vi "Default Success Response.vi"(8 "error in (no error)":errorcluster, 9 "Session In":refnum<class "Session.lvclass">, 10 "User":refnum<class "User.lvclass">) -> (0 "error out":errorcluster, 1 "Session":refnum<class "Session.lvclass">, 2 "Response":refnum<class "Response.lvclass">)   [LabVIEW 2020, in "HTTP Server.lvlib" / "Authentication Provider.lvclass"]
uses:
  Authentication Provider.lvclass
  lv-http-util/HTTP Utils/Response/Response.lvclass
  Session/Session.lvclass
  User/User.lvclass
  lv-http-util/HTTP Utils/Redirect Response/Redirect Response.lvclass
  C:/dev/lv20CE/relink/lv-http-util/HTTP Utils/Response/Response.lvclass
  lv-uri/URI/URI/URI.lvclass
  C:/dev/lv20CE/relink/lv-http-util/HTTP Utils/Redirect Response/Redirect Response.lvclass
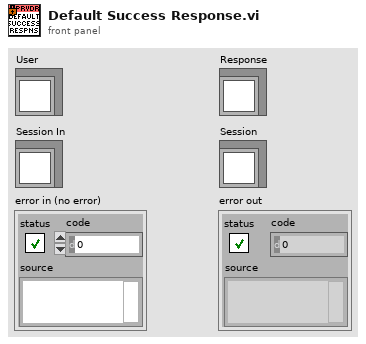
[diagram p1: front panel]
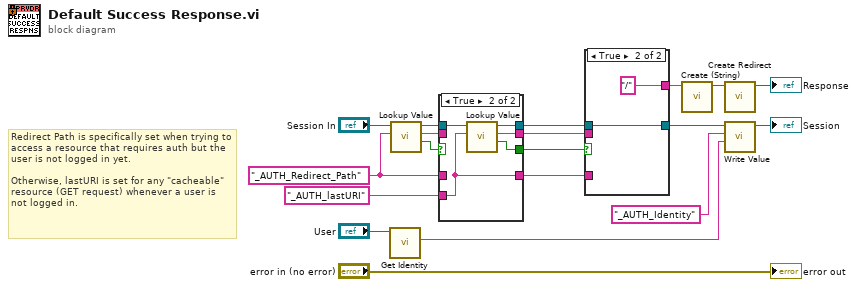
[diagram p0: block diagram]
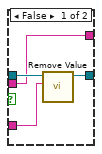
[diagram p2: hidden frame]
diagram:
  w7 = "_AUTH_Redirect_Path" ("Name")
  # "Redirect Path is specifically set when trying to access a resource that requires auth but the user is not logged in yet.\n\nOtherwise, lastURI is set for any \"cacheable\" resource (GET request) whenever a user is not logged in."
  n1 = call-dynamic "Get Identity.vi"("User in"="User") -> ("Identity"=w17:string)  [unwired: 8 in, 2 out]
  n2 = call "Lookup Value.vi"("Name"=w7, "Session in"="Session In") -> ("Not Found?"=w14:bool, "Value"=w12:string, "Session out"=w13:refnum<class "Session.lvclass">)  [unwired: 6 in, 1 out]
  n3 = case shown="True" w14 {
    tunnel: "_AUTH_lastURI" -> [_ w23]
    tunnel: w13 -> [w22 w27]
    tunnel: w12 -> [w21 _]
    tunnel: [_ w26] -> w9
    tunnel: [w21 w25] -> w10
    tunnel: [w22 w24] -> w11
    tunnel: [w20 w23] -> w8
    tunnel: w7 -> [w20 _]
    frame False {
    }
    frame True {
      n4 = call "Lookup Value.vi"("Name"=w23, "Session in"=w27) -> ("Not Found?"=w26:bool, "Value"=w25:string, "Session out"=w24:refnum<class "Session.lvclass">)  [unwired: 6 in, 1 out]
    }
  }
  n5 = case shown="True" w9 {
    tunnel: w11 -> [w29 w33]
    tunnel: w10 -> [w28 _]
    tunnel: [w28 "/" ("Value")] -> w6
    tunnel: [w30 w33] -> w5
    tunnel: w8 -> [w31 _]
    frame False {
      n6 = call "Remove Value.vi"("Name"=w31, "Session in"=w29) -> ("Session out"=w30:refnum<class "Session.lvclass">)  [unwired: 6 in, 3 out]
    }
    frame True {
    }
  }
  n7 = call "Create (String).vi"("URI String"=w6) -> ("URI out"=w16:refnum<class "URI.lvclass">)  [unwired: 9 in, 1 out]
  n8 = call "Create Redirect.vi"("Redirect URI"=w16) -> ("Redirect Response out"=→"Response":refnum<class "Redirect Response.lvclass">)  [unwired: 9 in, 1 out]
  n9 = call "Write Value.vi"("Value"=w17, "Name"="_AUTH_Identity", "Session in"=w5) -> ("Session out"=→"Session":refnum<class "Session.lvclass">)  [unwired: 6 in, 2 out]
  "error out" <- "error in (no error)"
